vi "OAT_Campbell Diagram_Locate Circles.vi"(4 "max circle overlap":dbl=0.4 format="%.2f", 6 "picture size (w,h)":cluster{"width":i16, "height":i16}, 7 "number of x steps":i32=12, 8 "Reference Level":dbl=10.0, 9 "y scale":cluster{"offset":dbl, "multiplier":dbl} {"multiplier" format="%.2f"; "offset" format="%.2f"}, 10 "x scale":cluster{"offset":dbl, "multiplier":dbl} {"multiplier" format="%.2f"; "offset" format="%.2f"}, 11 "map":dbl[][](array[numeric]) format="%.2f") -> (3 "circles":T1(array[cluster]) {"radius [pixel]" format="%.2f"; "y [EU]" format="%.2f"; "x [EU]" format="%.2f"})   [LabVIEW 2017]
uses:
  <vilib>/Analysis/1siggen.llb/Ramp Pattern by Samples.vi
  <vilib>/Analysis/NI_AALBase.lvlib
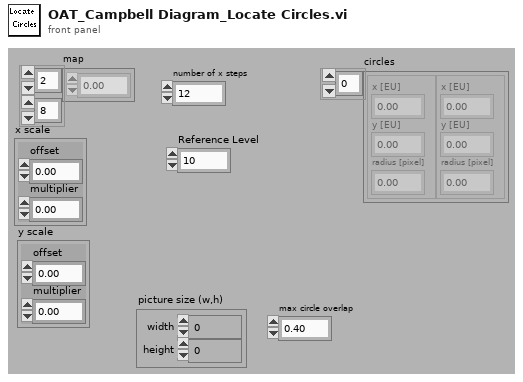
[diagram p1: front panel]
types:
  T1 = cluster{"x [EU]":dbl, "y [EU]":dbl, "radius [pixel]":dbl}[]
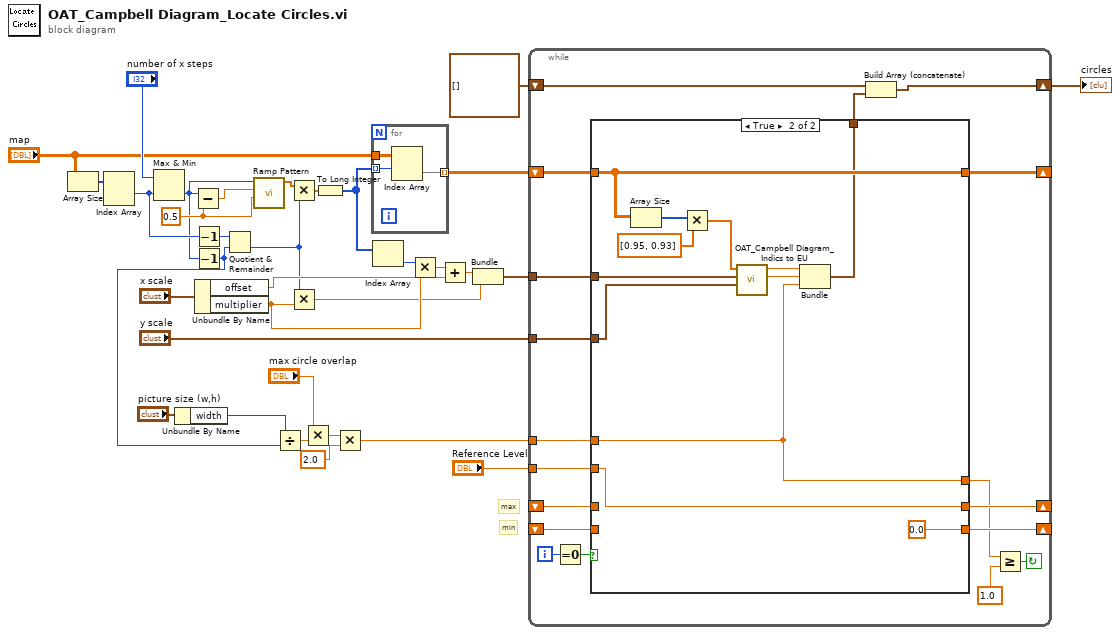
[diagram p0: block diagram]
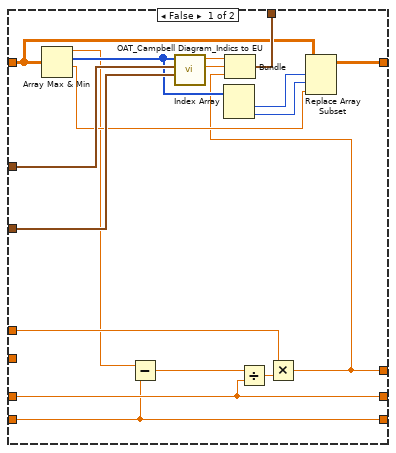
[diagram p2: hidden frame]
diagram:
  w26 = 0.5
  # "min"
  # "max"
  n1 = Array Size(array="map") -> (size(s)=w33:i32[])
  n2 = Index Array(array=w33) -> (element #1=w29:i32)  [unwired: 2 in, 1 out]
  n3 = Max & Min(x="number of x steps", y=w29) -> (min(x,y)=w24:i32)  [unwired: 1 out]
  n4 = Unbundle By Name("picture size (w,h)") -> ("width"=w2:i16)
  n5 = Subtract(x=w24, y=w26) -> (x-y=w25:dbl)
  n6 = Decrement(x=w29) -> (x-1=w28:i32)
  n7 = Decrement(x=w24) -> (x-1=w11:i32)
  n8 = Unbundle By Name("x scale") -> ("offset"=w17:dbl, "multiplier"=w19:dbl)
  n9 = Quotient & Remainder(x=w28, y=w11) -> (floor(x/y)=w3:i32)  [unwired: 1 out]
  n10 = call-poly <vilib>:"Ramp Pattern.vi"("start"=w26, "end"=w25, "samples"=w24) -> ("Ramp Pattern"=w23:dbl[])  [unwired: 7 in, 1 out]
  n11 = Divide(x=w2, y=w11) -> (x/y=w10:dbl)
  n12 = Multiply(x=w23, y=w3) -> (x*y=w27:dbl[])
  n13 = Multiply(x=w3, y=w19) -> (x*y=w15:dbl)
  n14 = Multiply(x="max circle overlap", y=w10) -> (x*y=w8:dbl)
  n15 = To Long Integer(number=w27) -> (32bit integer=w22:i32[])
  n16 = Multiply(x=w8, y=2.0) -> (x*y=w6:dbl)
  n17 = for {
    tunnel: "map" -> [w36]
    tunnel: w22 -> [w35] mode=indexing
    tunnel: [w34] -> w30 mode=indexing
    n18 = Index Array(array=w36, index (row)=w35) -> (element=w34:dbl[])  [unwired: 1 in]
  }
  n19 = Index Array(array=w22) -> (element=w20:i32)  [unwired: 1 in]
  n20 = Multiply(x=w20, y=w19) -> (x*y=w18:dbl)
  n21 = Add(x=w18, y=w17) -> (x+y=w16:dbl)
  n22 = Bundle(w16, w15) -> (w14:cluster{dbl, dbl})  [unwired: 1 in]
  n23 = while {
    shift-left: _ -> [w42]
    shift-right: [w43] -> _
    shift-left: cluster{"x [EU]":dbl, "y [EU]":dbl, dbl}[] [] -> [w46]
    shift-right: [w47] -> w4
    tunnel: w6 -> [w49]
    shift-left: _ -> [w50]
    shift-right: [w51] -> _
    tunnel: "y scale" -> [w52]
    tunnel: w14 -> [w53]
    shift-left: w30 -> [w45]
    shift-right: [w44] -> _
    tunnel: "Reference Level" -> [w41]
    i -> [w54]
    stop <- w37 continue-if-true
    n24 = Equal To 0?(x=w54) -> (x = 0?=w40:bool)
    n25 = case shown="True" w40 {
      tunnel: w53 -> [w72 w82]
      tunnel: w52 -> [w71 w83]
      tunnel: [w70 w74] -> w51
      tunnel: w50 -> [w70 _]
      tunnel: w49 -> [w69 w73]
      tunnel: [w66 w78] -> w48
      tunnel: w45 -> [w65 w81]
      tunnel: [w61 w81] -> w44
      tunnel: [w59 0.0] -> w43
      tunnel: w42 -> [w59 _]
      tunnel: w41 -> [_ w74]
      tunnel: [w55 w73] -> w38
      frame False {
        n26 = Array Max & Min(array=w65) -> (max value=w58:dbl, max index (indices)=w64:i32[], min value=w60:dbl)  [unwired: 1 out]
        n27 = Subtract(x=w58, y=w59) -> (x-y=w56:dbl)
        n28 = call <vilib>:"OAT_Campbell Diagram_Indics to EU.vi"("y scale"=w71, "x scale"=w72, "indices"=w64) -> ("y [EU]"=w67:dbl, "x [EU]"=w68:dbl)  [unwired: 7 in]
        n29 = Index Array(array=w64) -> (element #1=w63:i32, element #2=w62:i32)  [unwired: 2 in]
        n30 = Divide(x=w56, y=w70) -> (x/y=w57:dbl)
        n31 = Multiply(x=w69, y=w57) -> (x*y=w55:dbl)
        n32 = Bundle("x [EU]"=w68, "y [EU]"=w67, w55) -> (w66:cluster{"x [EU]":dbl, "y [EU]":dbl, dbl})  [unwired: 1 in]
        n33 = Replace Array Subset(array=w65, new element=w60, index (row)=w63, index (col)=w62) -> (w61:dbl[][])
      }
      frame True {
        n34 = Array Size(array=w81) -> (size(s)=w76:i32[])
        n35 = Multiply(x=w76, y=dbl[] [0.95, 0.93]) -> (x*y=w77:dbl[])
        n36 = call <vilib>:"OAT_Campbell Diagram_Indics to EU.vi"("y scale"=w83, "x scale"=w82, "indices"=w77) -> ("y [EU]"=w79:dbl, "x [EU]"=w80:dbl)  [unwired: 7 in]
        n37 = Bundle("x [EU]"=w80, "y [EU]"=w79, w73) -> (w78:cluster{"x [EU]":dbl, "y [EU]":dbl, dbl})  [unwired: 1 in]
      }
    }
    n38 = Build Array (concatenate)(w46, w48) -> (w47:cluster{"x [EU]":dbl, "y [EU]":dbl, dbl}[])
    n39 = Greater Or Equal?(x=w38, y=1.0) -> (x >= y?=w37:bool)
  }
  "circles" <- w4
